vi "Read Reader Model.vi"(0 "COM":refnum<visa-resource-name>, 1 "Timeout (ms)":u32=500, 7 "Address":string="01", 11 "error in (no error)":errorcluster) -> (4 "COM OUT":refnum<visa-resource-name>, 6 "ReceiveString":string, 15 "error out":errorcluster)   [LabVIEW 2020, in "Reader.lvlib"]
uses:
  Reader.lvlib
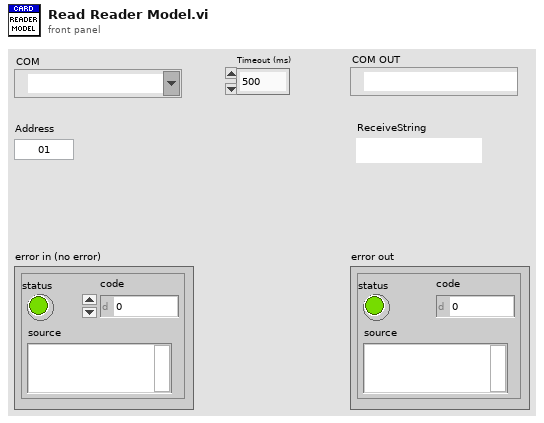
[diagram p1: front panel]
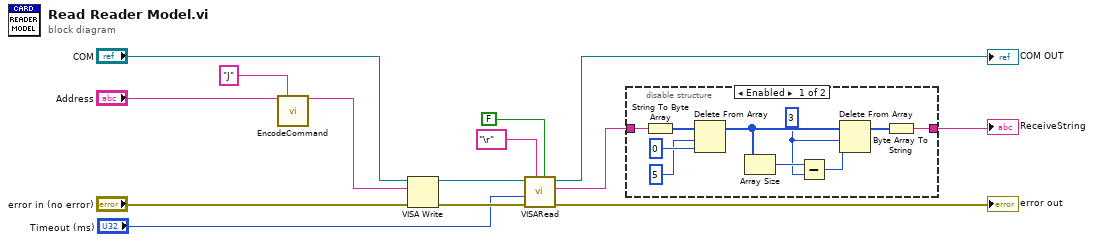
[diagram p0: block diagram]
diagram:
  n1 = call "EncodeCommand.vi"("Address"="Address", "Function"="J") -> ("Command String"=w9:string)  [unwired: 12 in, 1 out]
  n2 = VISA Write(VISA resource name="COM", write buffer=w9, error in (no error)="error in (no error)") -> (VISA resource name out=w11:refnum<visa-resource-name>, error out=w10:errorcluster)  [unwired: 1 out]
  n3 = call "VISARead.vi"("Delete Termination Char (False)"=FALSE, "Termination Char (blank)"="\r" ("Read regular"), "error in (no error)"=w10, "Timeout (ms)"="Timeout (ms)", "Resource in"=w11) -> ("error out"=→"error out":errorcluster, "Read Char"=w2:string, "Resource out"=→"COM OUT":refnum<visa-resource-name>)  [unwired: 4 in]
  n4 = disable-structure shown="Enabled" {
    disable-tunnel: w2 -> [w17 w25]
    disable-tunnel: [w16 w25] -> w1
    frame Enabled {
      w15 = 3 ("y")
      n5 = String To Byte Array(string=w17) -> (unsigned byte array=w24:u8[])
      n6 = Delete From Array(array=w24, length=5 ("length (len. of substring)"), index=0) -> (array with subset deleted=w22:u8[])  [unwired: 1 out]
      n7 = Array Size(array=w22) -> (size(s)=w21:i32)
      n8 = Subtract(x=w21, y=w15) -> (x-y=w19:i32)
      n9 = Delete From Array(array=w22, length=w15, index=w19) -> (array with subset deleted=w18:u8[])  [unwired: 1 out]
      n10 = Byte Array To String(unsigned byte array=w18) -> (string=w16:string)
    }
    frame Disabled {
    }
  }
  "ReceiveString" <- w1
